vi "ExampleAutoMessageFGV.vi"() -> ()   [LabVIEW 2019, in "MicronTemplateAPIs.lvlib" / "MicronTemplateAPIs.lvclass"]
uses:
  MicronTemplateAPIs.lvclass
  9ceadd3c-745e-4cc0-becc-c9896ef65399.vi
panel:
  out "Numeric3":dbl
  in  "Numeric2":dbl=2.0
  in  "Numeric1":dbl=42.0
  out "error out":errorcluster
  # "Here in this example, the inputs are not explicitly wired to the message API.\nThese are dynamically extracted, sent as message to the service and the output is \npopulated back in the UI.\n\nThe name of the VI and the list of controls names and data types in this client side example should exactly match the control names on the server API.\n\nRefer to MicronTemplateCore.lvclass\\Methods\\ExampleAutoMessageFGV.vi"
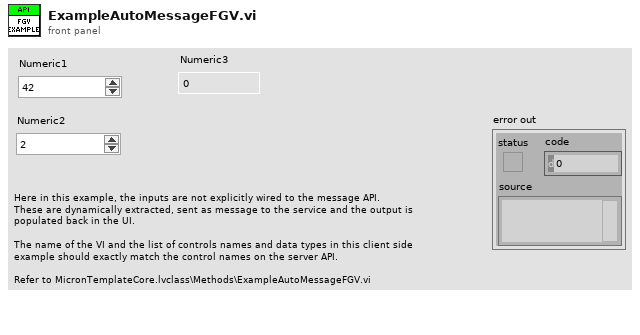
[diagram p1: front panel]
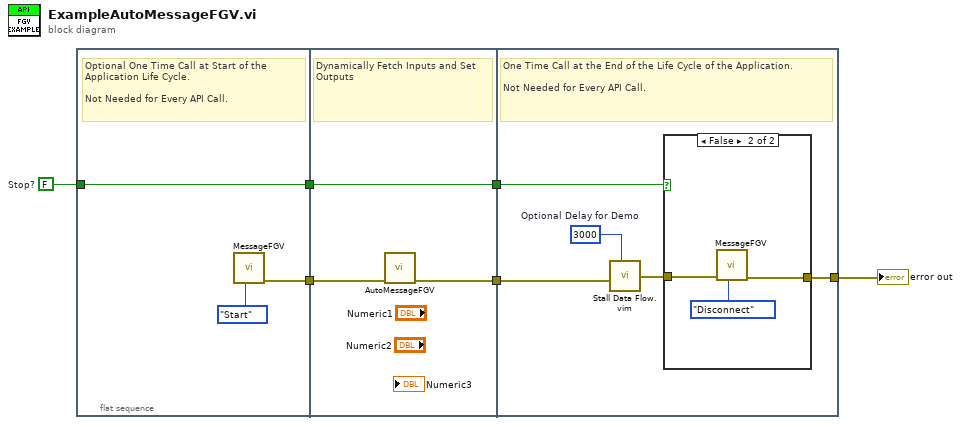
[diagram p0: block diagram]
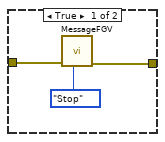
[diagram p2: hidden frame]
diagram:
  w1 = FALSE  # Stop?
  n1 = flat-sequence {
    tunnel: [w8] -> w4
    tunnel: [w7] -> w2
    tunnel: w1 -> [w7]
    tunnel: [w11] -> w5
    tunnel: w4 -> [w12]
    tunnel: [w10] -> w3
    tunnel: w2 -> [w10]
    tunnel: [w14] -> w6
    tunnel: w5 -> [w16]
    tunnel: w3 -> [w13]
    frame #0 {
      # "Optional One Time Call at Start of the Application Life Cycle.\n\nNot Needed for Every API Call."
      n2 = call "MessageFGV.vi"("Operation"=enum16{"Start", "Message", "Stop", "Disconnect"}."Start") -> ("error out"=w8:errorcluster)  [unwired: 9 in, 1 out]
    }
    frame #1 {
      # "Dynamically Fetch Inputs and Set Outputs"
      n3 = call "AutoMessageFGV.vi"("error in (no error)"=w12) -> ("error out"=w11:errorcluster)  [unwired: 9 in, 1 out]
    }
    frame #2 {
      w17 = u32 3000  # Optional Delay for Demo
      # "One Time Call at the End of the Life Cycle of the Application.\n\nNot Needed for Every API Call."
      n4 = call "Stall Data Flow.vim"("value in"=w16, "milliseconds to wait"=w17) -> ("value out"=w15:errorcluster)  [unwired: 1 out]
      n5 = case shown="False" w13 {
        tunnel: w15 -> [w20 w23]
        tunnel: [w19 w22] -> w14
        frame True {
          n6 = call "MessageFGV.vi"("Operation"=enum16{"Start", "Message", "Stop", "Disconnect"}."Stop", "error in (no error)"=w20) -> ("error out"=w19:errorcluster)  [unwired: 8 in, 1 out]
        }
        frame False {
          n7 = call "MessageFGV.vi"("Operation"=enum16{"Start", "Message", "Stop", "Disconnect"}."Disconnect", "error in (no error)"=w23) -> ("error out"=w22:errorcluster)  [unwired: 8 in, 1 out]
        }
      }
    }
  }
  "error out" <- w6
